vi "configure.vi"(8 "error in (no error)":errorcluster, 11 "GenericPlugin in":refnum<class "StageMMS2015ASIfromScientifica.lvclass">) -> (0 "error out":errorcluster, 3 "GenericPlugin out":refnum<class "StageMMS2015ASIfromScientifica.lvclass">)   [LabVIEW 2010, in "StageMMS2015ASIfromScientifica.lvclass"]
doc: "The dynamic dispatch version of this VI loads and displays the configuration file associated with the plug-in object. The user modify and save the configuration data."
uses:
  StageMMS2015ASIfromScientifica.lvclass
  StageMMS2015ASIfromScientifica.lvclass/StageMMS2015ASIfromScientifica.ctl
  common/classes/GenericComponent/GenericComponent/GenericComponent.lvclass
panel:
  in  "serial port name":refnum<visa-resource-name>
  out "configuration":string
  in  "cancelButton":bool
  in  "okButton":bool
  # "Configure MH110930Scientifica"
  # "settings"
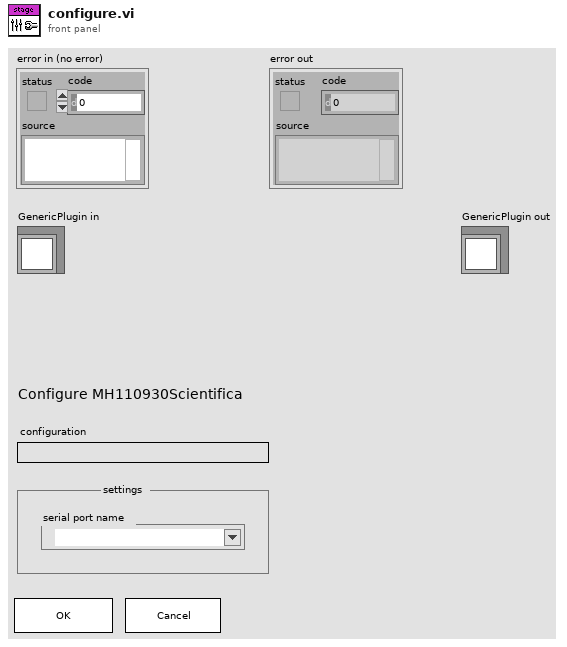
[diagram p1: front panel]
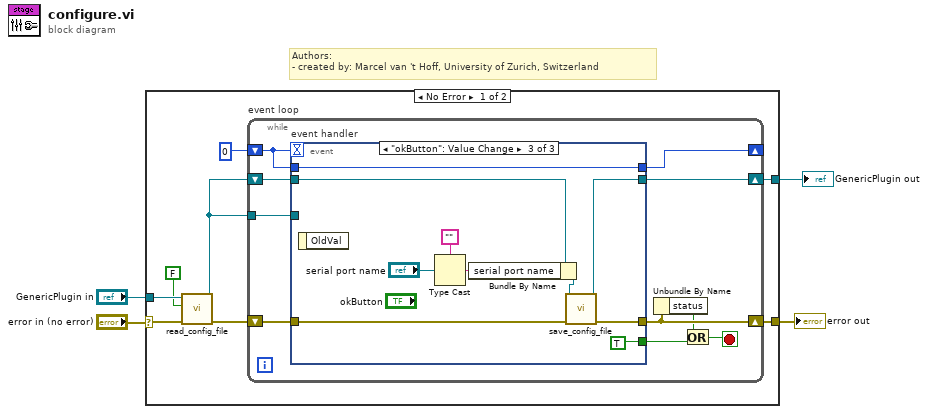
[diagram p0: block diagram]
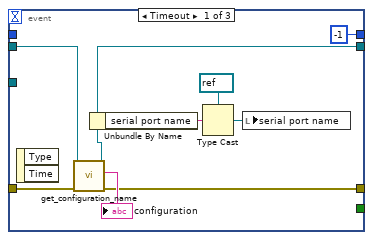
[diagram p2: hidden frame]
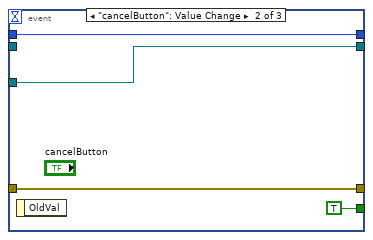
[diagram p3: hidden frame]
diagram:
  # "Authors: \n- created by: Marcel van 't Hoff, University of Zurich, Switzerland"
  n1 = case shown="No Error" "error in (no error)" {
    selector: "error in (no error)" -> [w10 w46]
    tunnel: [w12 w46] -> w3
    tunnel: "GenericPlugin in" -> [w8 w47]
    tunnel: [w11 w47] -> w1
    frame No Error {
      n2 = call-dynamic "read_config_file.vi"("error in (no error)"=w10, "force load?"=FALSE, "GenericPlugin in"=w8) -> ("error out"=w9:errorcluster, "GenericPlugin out"=w5:refnum<class "StageMMS2015ASIfromScientifica.lvclass">)  [unwired: 7 in]
      n3 = while "event loop" {
        shift-right: [w19] -> w12
        shift-left: w9 -> [w22]
        shift-right: [w20] -> w11
        shift-left: w5 -> [w21]
        tunnel: w5 -> [w15]
        shift-right: [w13] -> _
        shift-left: 0 -> [w14]
        stop <- w16 stop-if-true
        n4 = event "event handler" shown="[2] \"okButton\": Value Change" {
          selector: _ -> [_ _ _]
          dyn-events: _ -> [_ _ _]
          timeout: w14 -> [_ _ _]
          tunnel: w22 -> [w31 w35 w39]
          tunnel: [w26 w35 w44] -> w19
          tunnel: w21 -> [w30 _ w41]
          tunnel: [w27 w33 w43] -> w20
          tunnel: [_ TRUE TRUE] -> w18
          tunnel: w15 -> [_ w33 _]
          tunnel: [-1 w32 w42] -> w13
          tunnel: w14 -> [_ w32 w42]
          event Timeout {
            n5 = event-data() -> ()  [unwired: 1 in, 2 out]
            n6 = call "get_configuration_name.vi"("error in (no error)"=w31, "GenericPlugin.lvclass in"=w30) -> ("error out"=w26:errorcluster, "configuration name"=→"configuration":string, "GenericPlugin.lvclass out"=w27:refnum<class "StageMMS2015ASIfromScientifica.lvclass">)  [unwired: 7 in]
            n7 = Unbundle By Name(w27) -> ("serial port name"=w25:string)
            n8 = Type Cast(type=refnum<visa-resource-name> refnum ("serial port name"), x=w25) -> (*(type *) &x=w23:refnum<visa-resource-name>)
            n9 = local write "serial port name"(w23) -> ()
          }
          event "cancelButton": Value Change {
            n10 = event-data() -> ()  [unwired: 1 in, 1 out]
          }
          event "okButton": Value Change {
            n11 = event-data() -> ()  [unwired: 1 in, 1 out]
            n12 = Type Cast(type="", x="serial port name") -> (*(type *) &x=w36:string)
            n13 = Bundle By Name(cluster=w41, "serial port name"=w36) -> (w40:refnum<class "StageMMS2015ASIfromScientifica.lvclass">)
            n14 = call-dynamic "save_config_file.vi"("error in (no error)"=w39, "GenericPlugin in"=w40) -> ("error out"=w44:errorcluster, "GenericPlugin out"=w43:refnum<class "StageMMS2015ASIfromScientifica.lvclass">)  [unwired: 8 in]
          }
        }
        n15 = Unbundle By Name(w19) -> ("status"=w17:bool)
        n16 = Or(x=w17, y=w18) -> (x .or. y?=w16:bool)
      }
    }
    frame Error {
    }
  }
  "error out" <- w3
  "GenericPlugin out" <- w1
